vi "KobukiOdometers.vi"(6 "ResetOdo":bool, 11 "Kobuki Sensors  in":T1) -> (0 "Accumulator":i16, 1 "Accumulator 2":i16, 2 "NetAngle":dbl, 3 "NetDistance":dbl)   [LabVIEW 2014]
uses:
  Kobuki/KobukiSensors.ctl
  Kobuki/Kobuki Bumps and WheelDrops.ctl
  Kobuki/Kobuki Buttons.ctl
  Kobuki/Charging Sources Available.ctl
panel:
  # "Electrical: charging, battery, OI mode"
  # "Sensors: bump, cliff, button, wheel drop, wall, virtual wall"
  # "Motors:"
  # "Song"
  # "Inertia"
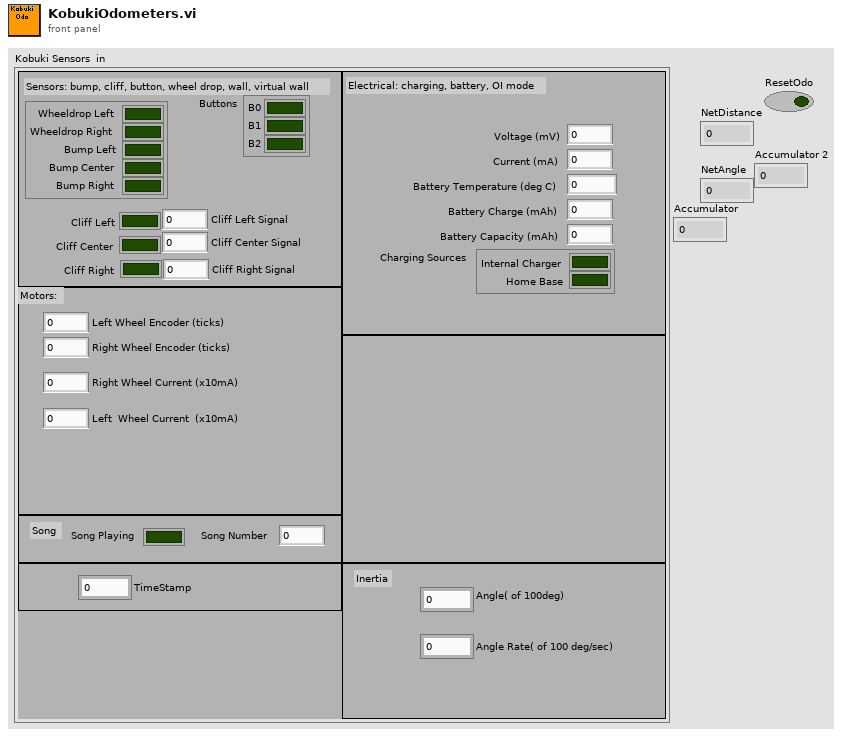
[diagram p1: front panel]
types:
  T1 = typedef "KobukiSensors.ctl" = cluster{"Bumps + Wheel Drops":T2, "Cliff Left":bool, "Cliff Center":bool, "Cliff Right":bool, "Cliff Left Signal":u16, "Cliff Center Signal":u16, "Cliff Right Signal":u16, "Buttons":T3, "Left Wheel Encoder (ticks)":u16, "Right Wheel Encoder (ticks) ":u16, "Right Wheel Current (x10mA)":i16, "Left  Wheel Current  (x10mA)":i16, "TimeStamp":u16, "Song Playing":bool, "Song Number":u8, "Voltage (mV)":i16, "Current (mA)":i16, "Battery Temperature (deg C)":i16, "Battery Charge (mAh)":i16, "Battery Capacity (mAh)":i16, "Charging Sources":T4, "Angle( of 100deg)":i16, "Angle Rate( of 100 deg/sec)":i16}
  T2 = typedef "Kobuki Bumps and WheelDrops.ctl" = cluster{"Wheeldrop Left":bool, "Wheeldrop Right":bool, "Bump Left":bool, "Bump Center":bool, "Bump Right":bool}
  T3 = typedef "Kobuki Buttons.ctl" = cluster{"B0":bool, "B1":bool, "B2":bool}
  T4 = typedef "Charging Sources Available.ctl" = cluster{"Internal Charger":bool, "Home Base":bool}
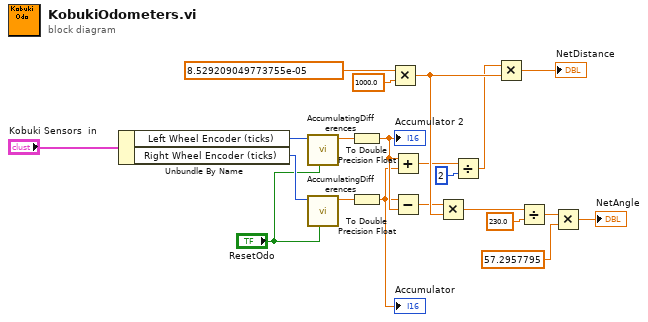
[diagram p0: block diagram]
diagram:
  n1 = Unbundle By Name("Kobuki Sensors  in") -> ("Left Wheel Encoder (ticks)"=w8:u16, "Right Wheel Encoder (ticks)"=w20:u16)
  n2 = call "AccumulatingDifferences.vi"("Reset"="ResetOdo", "input"=w8) -> ("Accumulator"=w19:dbl)  [unwired: 9 in]
  n3 = call "AccumulatingDifferences.vi"("Reset"="ResetOdo", "input"=w20) -> ("Accumulator"=w21:dbl)  [unwired: 9 in]
  n4 = To Double Precision Float(number=w19) -> (double precision float=w2:dbl)
  "Accumulator 2" <- w2
  n5 = To Double Precision Float(number=w21) -> (double precision float=w1:dbl)
  "Accumulator" <- w1
  n6 = Multiply(x=8.529209049773755e-05, y=1000.0) -> (x*y=w14:dbl)
  n7 = Add(x=w2, y=w1) -> (x+y=w9:dbl)
  n8 = Subtract(x=w1, y=w2) -> (x-y=w3:dbl)
  n9 = Multiply(x=w3, y=w14) -> (x*y=w15:dbl)
  n10 = Divide(x=w9, y=i16 2) -> (x/y=w11:dbl)
  n11 = Multiply(x=w11, y=w14) -> (x*y=→"NetDistance":dbl)
  n12 = Divide(x=w15, y=230.0) -> (x/y=w17:dbl)
  n13 = Multiply(x=w17, y=57.2957795) -> (x*y=→"NetAngle":dbl)
